vi "Settings Init.vi"(7 "Refs":T8, 8 "error in (no error)":errorcluster, 10 "Active Tag":string="Icon Editor", 11 "Data in":T1={"Class"={"Ants"=refnum, "Layer"=refnum, "Templates"=refnum, "Icon"=refnum, "Glyph"=refnum, "Settings"=refnum, "Tools"=refnum, "History"=refnum}, "Ref"={"Add Layer"=refnum, "Remove Layer"=refnum, "Line Text"=[], "Body Text Spec"=refnum, "DNL_Font"=refnum, "glyph path str"=refnum, "templates path str"=refnum, "Arrow Up"=refnum, "Arrow Down"=refnum, "IE VI Ref"=refnum, "Glyphs tree"=refnum, "Templates tree"=refnum, "Layer Icon Text"=refnum, "Layer Template"=refnum, "Body Text"=refnum, "Search Templates"=refnum, "TextMarker"=refnum, "Tab Control"=refnum, "Search Glyphs"=refnum, "Line Color"=refnum, "DNL_Glyphs []"=refnum, "Fill Color"=refnum, "Tools"=refnum, "Icon"=refnum, "Preview"=refnum, "Ants"=refnum, "Terminals"=refnum, "menu reference"=refnum, "LayerNames"=[], "GlyphLoadAnimation"=refnum, "TemplateLoadAnimation"=refnum, "refreshGlyphs"=refnum, "refreshTemplates"=refnum}, "Support"={"AntsRect"={"left"=0, "top"=0, "right"=0, "bottom"=0}, "Mouse Move Coords"={"Horizontal"=0, "Vertical"=0}, "Mouse Down Coords"={"Horizontal"=0, "Vertical"=0}, "Temp Coord"={"Horizontal"=0, "Vertical"=0}, "Action"=enum."Default", "Edge Color"=4914962, "Fill Color"=16860, "Mouse Down?"=FALSE, "Draft Mode?"=FALSE, "Temp Icon"=bytes[3102], "CTRL Pressed"=FALSE, "Move Selection?"=FALSE, "AntsRect Orig"={"left"=0, "top"=0, "right"=0, "bottom"=0}, "Text"="", "TM Set?"=FALSE, "Mouse inside icon?"=FALSE, "Tool (old value)"=0, "Pencil Move Color"=0, "Swap Colors?"=FALSE, "Shift pressed?"=FALSE}}) -> (0 "error out":errorcluster, 3 "Data out":T1={"Class"={"Ants"=refnum, "Layer"=refnum, "Templates"=refnum, "Icon"=refnum, "Glyph"=refnum, "Settings"=refnum, "Tools"=refnum, "History"=refnum}, "Ref"={"Add Layer"=refnum, "Remove Layer"=refnum, "Line Text"=[], "Body Text Spec"=refnum, "DNL_Font"=refnum, "glyph path str"=refnum, "templates path str"=refnum, "Arrow Up"=refnum, "Arrow Down"=refnum, "IE VI Ref"=refnum, "Glyphs tree"=refnum, "Templates tree"=refnum, "Layer Icon Text"=refnum, "Layer Template"=refnum, "Body Text"=refnum, "Search Templates"=refnum, "TextMarker"=refnum, "Tab Control"=refnum, "Search Glyphs"=refnum, "Line Color"=refnum, "DNL_Glyphs []"=refnum, "Fill Color"=refnum, "Tools"=refnum, "Icon"=refnum, "Preview"=refnum, "Ants"=refnum, "Terminals"=refnum, "menu reference"=refnum, "LayerNames"=[], "GlyphLoadAnimation"=refnum, "TemplateLoadAnimation"=refnum, "refreshGlyphs"=refnum, "refreshTemplates"=refnum}, "Support"={"AntsRect"={"left"=0, "top"=0, "right"=0, "bottom"=0}, "Mouse Move Coords"={"Horizontal"=0, "Vertical"=0}, "Mouse Down Coords"={"Horizontal"=0, "Vertical"=0}, "Temp Coord"={"Horizontal"=0, "Vertical"=0}, "Action"=enum."Default", "Edge Color"=4914962, "Fill Color"=16860, "Mouse Down?"=FALSE, "Draft Mode?"=FALSE, "Temp Icon"=bytes[3102], "CTRL Pressed"=FALSE, "Move Selection?"=FALSE, "AntsRect Orig"={"left"=0, "top"=0, "right"=0, "bottom"=0}, "Text"="", "TM Set?"=FALSE, "Mouse inside icon?"=FALSE, "Tool (old value)"=0, "Pencil Move Color"=0, "Swap Colors?"=FALSE, "Shift pressed?"=FALSE}})   [LabVIEW 2020]
uses:
  Class/Ants/Ants.lvclass
  Class/FakedArray/FakedArray.lvclass
  vi.lib/LabVIEW Icon API/lv_icon/Classes/Icon/Icon.lvclass
  Class/Icon Library/Glyph.lvclass
  Class/Settings/Settings.lvclass
  Class/Tools/Tools Paint.lvclass
  lv_icon.lvlib
  Controls/Settings.ctl
  <vilib>/Utility/miscctls.llb/LVPoint32TypeDef.ctl
  Controls/SupportClass_Action.ctl
  vi.lib/LabVIEW Icon API/lv_icon/Controls/IEColor.ctl
  Controls/Support Cluster.ctl
  Controls/References Cluster.ctl
  Controls/IE Classes.ctl
  Controls/Global Data.ctl
  History/History/History.lvclass
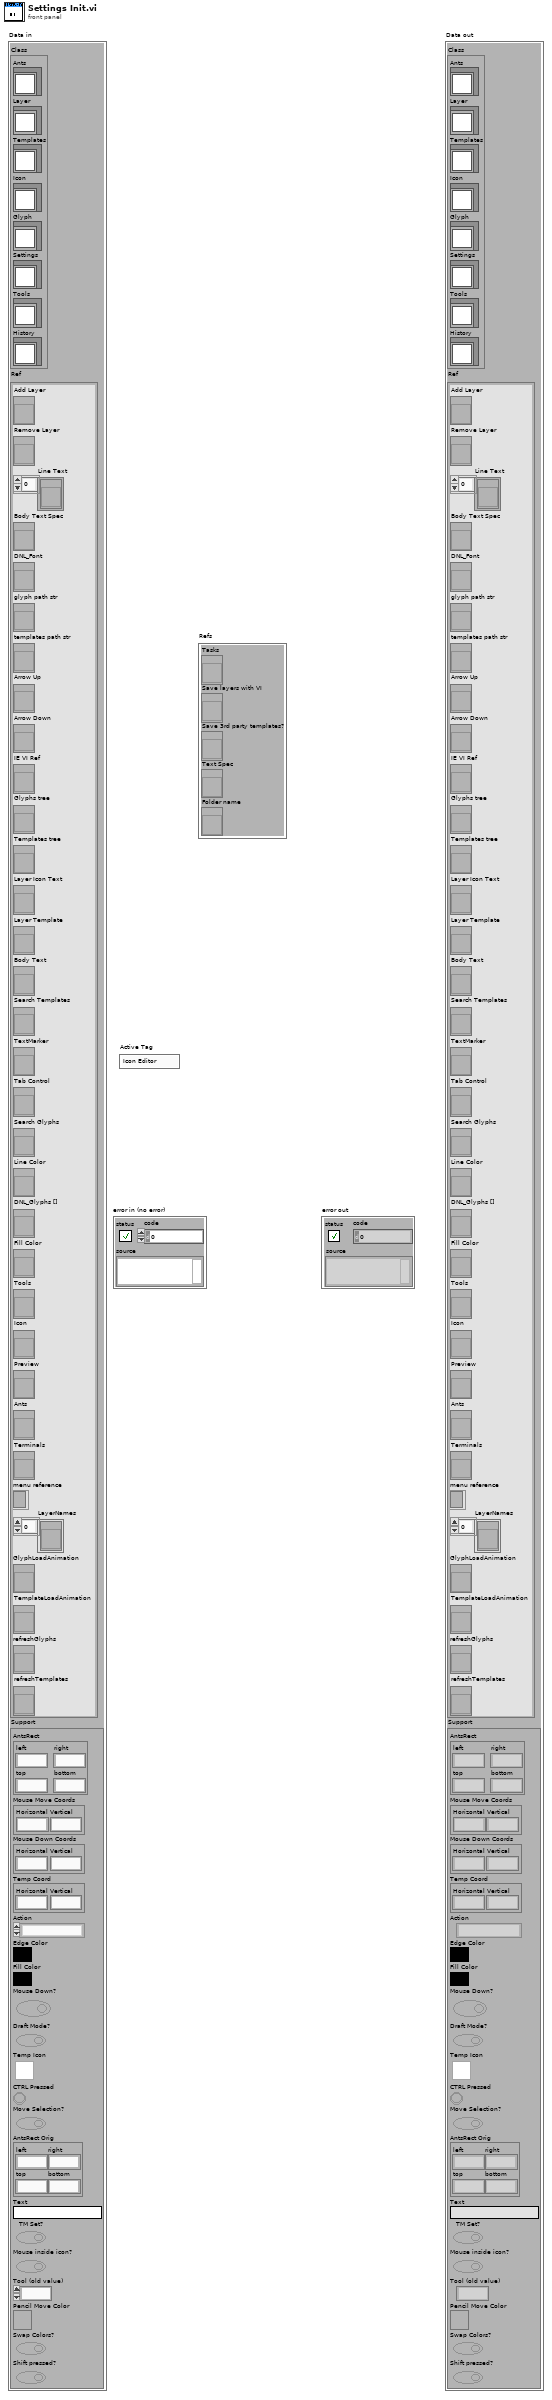
[diagram p1: front panel]
types:
  T1 = typedef "lv_icon.lvlib/Global Data.ctl" = cluster{"Class":T2, "Ref":T3, "Support":T4}
  T2 = typedef "lv_icon.lvlib/IE Classes.ctl" = cluster{"Ants":refnum<class "Ants.lvclass">, "Layer":refnum<class "FakedArray.lvclass">, "Templates":refnum<class "FakedArray.lvclass">, "Icon":refnum<class "Icon.lvclass">, "Glyph":refnum<class "Glyph.lvclass">, "Settings":refnum<class "Settings.lvclass">, "Tools":refnum<class "Tools Paint.lvclass">, "History":refnum<class "History.lvclass">}
  T3 = typedef "lv_icon.lvlib/References Cluster.ctl" = cluster{"Add Layer":refnum<vi>, "Remove Layer":refnum<vi>, "Line Text":refnum<vi>[], "Body Text Spec":refnum<vi>, "DNL_Font":refnum<vi>, "glyph path str":refnum<vi>, "templates path str":refnum<vi>, "Arrow Up":refnum<vi>, "Arrow Down":refnum<vi>, "IE VI Ref":refnum<vi>, "Glyphs tree":refnum<vi>, "Templates tree":refnum<vi>, "Layer Icon Text":refnum<vi>, "Layer Template":refnum<vi>, "Body Text":refnum<vi>, "Search Templates":refnum<vi>, "TextMarker":refnum<vi>, "Tab Control":refnum<vi>, "Search Glyphs":refnum<vi>, "Line Color":refnum<vi>, "DNL_Glyphs []":refnum<vi>, "Fill Color":refnum<vi>, "Tools":refnum<vi>, "Icon":refnum<vi>, "Preview":refnum<vi>, "Ants":refnum<vi>, "Terminals":refnum<vi>, "menu reference":refnum<k9>, "LayerNames":refnum<vi>[], "GlyphLoadAnimation":refnum<vi>, "TemplateLoadAnimation":refnum<vi>, "refreshGlyphs":refnum<vi>, "refreshTemplates":refnum<vi>}
  T4 = typedef "lv_icon.lvlib/Support Cluster.ctl" = cluster{"AntsRect":cluster{"left":i16, "top":i16, "right":i16, "bottom":i16}, "Mouse Move Coords":T5, "Mouse Down Coords":T5, "Temp Coord":T5, "Action":T6, "Edge Color":T7, "Fill Color":T7, "Mouse Down?":bool, "Draft Mode?":bool, "Temp Icon":picture, "CTRL Pressed":bool, "Move Selection?":bool, "AntsRect Orig":cluster{"left":i16, "top":i16, "right":i16, "bottom":i16}, "Text":string, "TM Set?":bool, "Mouse inside icon?":bool, "Tool (old value)":u32, "Pencil Move Color":u32, "Swap Colors?":bool, "Shift pressed?":bool}
  T5 = typedef "LVPoint32TypeDef.ctl" = cluster{"Horizontal":i32, "Vertical":i32}
  T6 = typedef "SupportClass_Action.ctl" = enum16{"Default", "Move Selection", "Glyph Library", "Tool"}
  T7 = typedef "IEColor.ctl" = u32
  T8 = typedef "Settings.ctl" = cluster{"Tasks":refnum<vi>, "Save layers with VI":refnum<vi>, "Save 3rd party templates?":refnum<vi>, "Text Spec":refnum<vi>, "Folder name":refnum<vi>}
  T9 = typedef "Font.ctl" = string
  T10 = typedef "Alignment.ctl" = u16
  T11 = typedef "Font Size.ctl" = u8
  T12 = typedef "Who Invoked Icon Editor.ctl" = cluster{"Icon Editor Invoker Type":T13, "App Refnum of Invoker":refnum<vi>, "Qualified Name of Invoker":string, "Path to Invoker":path}
  T13 = typedef "Icon Editor Invoker Type.ctl" = enum32{"Unknown Icon Source", "VI Icon", "Library Icon (any library type)", "Palette icon", "Icon from App Method"}
  T14 = cluster{"Same Folder Structure?":bool, "Folder Name":string}
  T15 = typedef "Pathes.ctl" = enum16{"Root Path", "Icon Templates", "Icon Templates VI", "Icon Templates Lib", "Glyphs"}
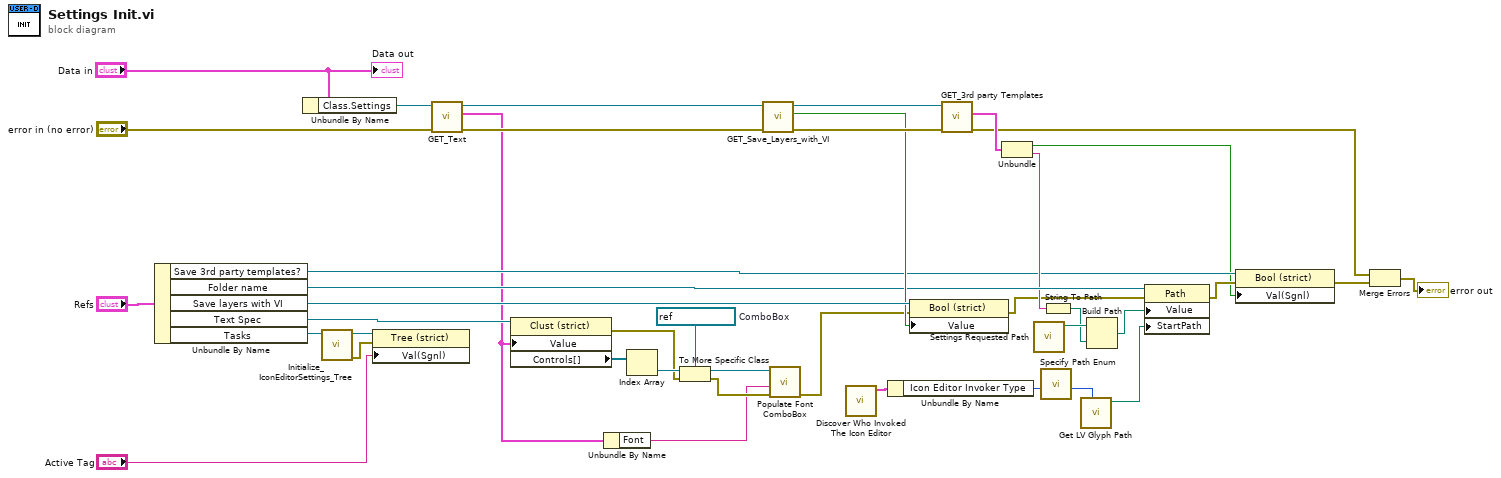
[diagram p0: block diagram]
diagram:
  w13 = refnum<vi> refnum  # ComboBox
  n1 = Unbundle By Name("Refs") -> ("Save 3rd party templates?"=w28:refnum<vi>, "Folder name"=w31:refnum<vi>, "Save layers with VI"=w34:refnum<vi>, "Text Spec"=w35:refnum<vi>, "Tasks"=w21:refnum<vi>)
  n2 = Unbundle By Name("Data in") -> ("Class.Settings"=w4:refnum<class "Settings.lvclass">)
  n3 = call "Initialize_IconEditorSettings_Tree.vi"("Tree Refnum"=w21) -> ("error out"=w20:errorcluster)  [unwired: 1 in, 9 out]
  n4 = property class="Tree (strict)"(reference=w21, error in=w20, "Val(Sgnl)"="Active Tag") -> ()  [unwired: 2 out]
  n5 = call-dynamic "GET_Text.vi"("error in (no error)"="error in (no error)", "Settings.lvclass in"=w4) -> ("error out"=w38:errorcluster, "Text"=w10:cluster{"Font":T9, "Alignment":T10, "Size":T11}, "Settings.lvclass out"=w37:refnum<class "Settings.lvclass">)  [unwired: 7 out]
  n6 = property class="Clust (strict)"(reference=w35, "Value"=w10) -> (error out=w14:errorcluster, "Controls[]"=w16:refnum<vi>[])  [unwired: 1 in, 1 out]
  n7 = Unbundle By Name(w10) -> ("Font"=w9:T9)
  n8 = Index Array(array=w16) -> (element=w15:refnum<vi>)  [unwired: 1 in]
  n9 = To More Specific Class(target class=w13, reference=w15, error in=w14) -> (specific class reference=w12:refnum<vi>, error out=w11:errorcluster)
  n10 = call "GET_Save_Layers_with_VI.vi"("error in (no error)"=w38, "Settings.lvclass in"=w37) -> ("error out"=w39:errorcluster, "Merge user layers on commit"=w33:bool, "Settings.lvclass out"=w40:refnum<class "Settings.lvclass">)  [unwired: 7 out]
  n11 = call "Populate Font ComboBox.vi"("error in"=w11, "Font in"=w9, "CmbBox Refnum"=w12) -> ("error out"=w8:errorcluster)  [unwired: 8 out]
  n12 = call <resource>:"Discover Who Invoked The Icon Editor.vi"() -> ("Who Invoked The Icon Editor?"=w23:T12)  [unwired: 11 out]
  n13 = Unbundle By Name(w23) -> ("Icon Editor Invoker Type"=w7:T13)
  n14 = property class="Bool (strict)"(reference=w34, error in=w8, "Value"=w33) -> (error out=w29:errorcluster)  [unwired: 1 out]
  n15 = call-dynamic "GET_3rd party Templates.vi"("error in (no error)"=w39, "Settings.lvclass in"=w40) -> ("error out"=w2:errorcluster, "3rd party Templates"=w32:T14)  [unwired: 8 out]
  n16 = Unbundle(w32) -> ("Same Folder Structure?"=w26:bool, "Folder Name"=w30:string)
  n17 = call "Settings Requested Path.vi"() -> ("Requested Path"=w19:path)  [unwired: 11 out]
  n18 = call "Specify Path Enum.vi"("Icon Editor Invoker Type"=w7) -> ("Path"=w6:T15)  [unwired: 10 out]
  n19 = String To Path(string=w30) -> (path=w18:path)
  n20 = call "Get LV Glyph Path.vi"("Path"=w6) -> ("Requested Path"=w22:path)  [unwired: 2 in, 8 out]
  n21 = Build Path(base path=w19, name or relative path=w18) -> (appended path=w17:path)
  n22 = property class="Path"(reference=w31, error in=w29, "Value"=w17, "StartPath"=w22) -> (error out=w27:errorcluster)  [unwired: 1 out]
  n23 = property class="Bool (strict)"(reference=w28, error in=w27, "Val(Sgnl)"=w26) -> (error out=w1:errorcluster)  [unwired: 1 out]
  n24 = Merge Errors(w2, w1) -> (→"error out":errorcluster)
  "Data out" <- "Data in"
